vi "pruebaMaquinaEstados.vi"() -> ()   [LabVIEW 2016]
uses:
  Control 1.ctl
  <vilib>/userdefined/High Color/IMAQdx.ctl
  <vilib>/vision/driver/NI_Vision_Acquisition_Software.lvlib
panel:
  in  "Guardado":bool
  in  "D 4":i32
  in  "I 3":i32
  in  "I 2":i32
  in  "I 1":i32
  in  "D 3":i32
  in  "D 2":i32
  in  "D 1":i32
  in  "Movimiento de spot en x":ext(slide)=0.5255 scale=-10.0..10.0
  in  "Movimiento de spot en y":dbl(slide)=0.78 min=-10.0 max=10.0 scale=-10.0..10.0
  in  "Gráficas visibles":bool[](array[boolean])=[FALSE, FALSE, TRUE, FALSE, FALSE, FALSE]
  in  "Ver cámara":bool
  out "Image Pixels (U8)":u8[][](array[numeric])
  out "espectro aeereglo":dbl[][](array[numeric])
  in  "Cancel Button":bool
  in  "Guardar":bool=TRUE
  in  "valor delay":u32=300
  in  "tiempo de delay":u32=300
  out "Orden":T1(array[ring])=[enum."espejos", enum."voltaje", enum."polarizador", enum."potenciometro ", enum."CCD"]
  in  "Nombre  archivo":string="prueba0404"
  in  "stop medición":bool
  in  "stop":bool
  in  "Iniciar medición":bool
  out "Control de espejos":T2={"Movimiento de spot en y"=0.78, "Movimiento de spot en x"=0.5255, "tipo "=enum."barrido", "yFin"=0.82, "Paso"=0.01, "xFin"=0.5655} {"Movimiento de spot en x" scale=-10.0..10.0; "Movimiento de spot en y" min=-10.0 max=10.0 scale=-10.0..10.0}
  out "Config. voltaje y corriente":T3 {"Measurement Function (0:Voltage)" items=["Voltage", "Current", "Power"]; "Unit(V)" items=["V", "mV", "kV", "A", "mA"]; "Function(0:Voltage)" items=["Voltage", "Current"]}
  out "Laser":T4
  out "Config. fotodiodo y potenciometro":T5={"tiempo. lect."=300, "num. med"=20, "tiempo. lectura"=0, "average rate"=0, "Readout Config"="POW", "Tipo de Medición"=enum."Lockin", "usar multimetro"=FALSE}
  out "Control CCD":T6={"Numero de lecturas"=0, "tiempo de lectura (ms)"=100, "Exposure"=0.053229, "Valor Gamma"=1.0, "Ganancia"=33, "Opción"=enum."Espectro", "VISA resource name"="", "Enable Strobe (Disabled)"=FALSE} {"Ganancia" min=0 max=100; "Valor Gamma" min=1.0 max=2.2; "Exposure" min=5e-05 max=0.053229}
  out "config. Polarizador":T7={"pos inic"=0.0, "pos.final"=5.0, "incremento"=1.0, "velocidad"=0.0}
  in  "medir corriente":bool
  out "xsal":dbl=-0.20408163265306034
  out "ysal":dbl
  out "Ángulo del polarizador":dbl=5.000014648473263
  out "corriente":dbl
  out "voltaje":dbl
  out "temperatura":dbl
  out "corriente laser":dbl
  out "multimetro":dbl
  out "valor potenciometro":dbl=nan format="%^#_9e"
  out "LockIn":dbl=0.0003
  out "multímetro":T8
  out "Dr/r":T8
  out "espectro":T8={[0.0, 1.0, 2.0000073242366314, 3.0000073242366314, 4.000007324236631, 5.000014648473263], [0.0003, 0.0003, 0.0003, 0.0003, 0.0003, 0.0003]}
  out "I-V":cluster{dbl[], dbl[]}(graph)
  out "Gráfica general":T8={[0.0, 1.0, 2.0000073242366314, 3.0000073242366314, 4.000007324236631, 5.000014648473263], [0.0003, 0.0003, 0.0003, 0.0003, 0.0003, 0.0003]}
  out "Power meter":cluster{dbl[], dbl[]}(graph)
  out "Imágen":T9(plugin-control)
  in  "SerialNumber":string="55000538"
  # "Gráfica general"
  # "Gráfica potenciómetro"
  # "Gráfica I-V"
  # "Control espejos"
  # "Multímetro"
  # "División"
  # "Espectro"
  # "Amplificador Lock in"
  # "potenciometro"
  # "Espectro"
  # "Imágen"
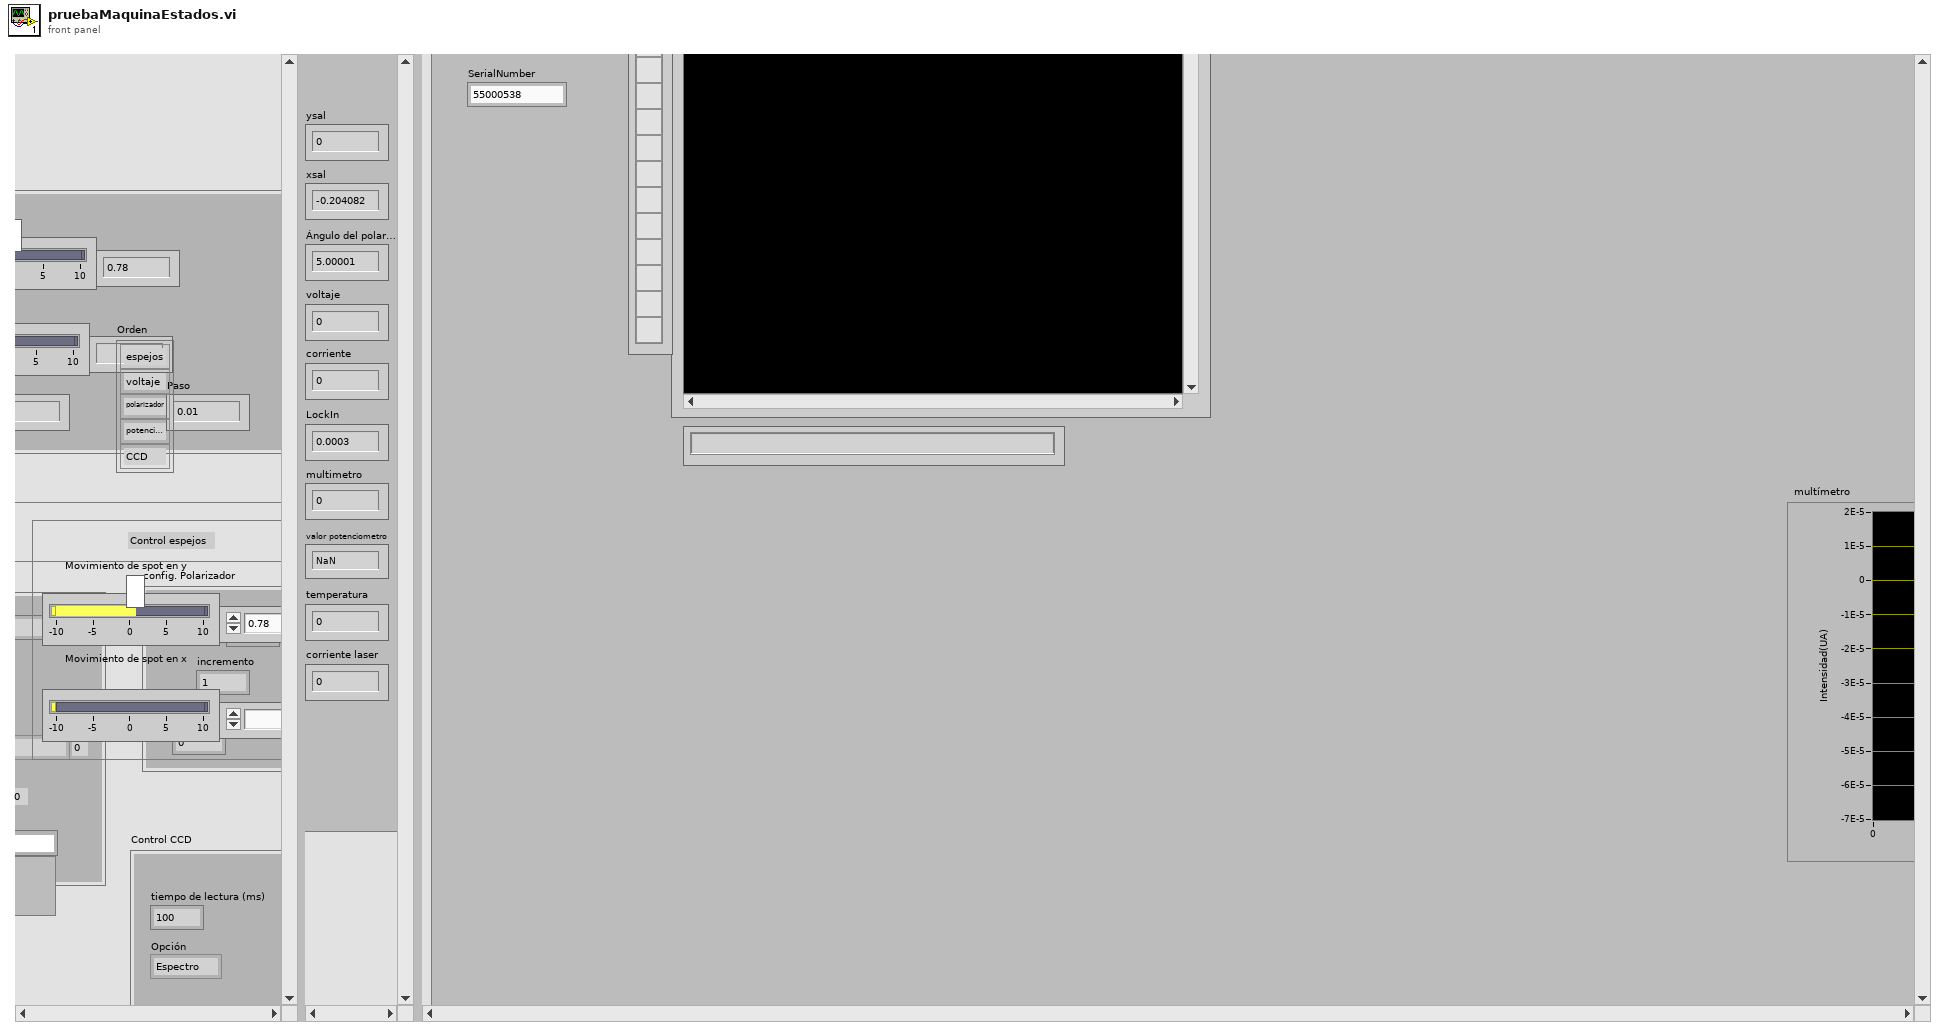
[diagram p1: front panel]
types:
  T1 = enum16{"espejos", "polarizador", "voltaje", "potenciometro ", "CCD", "lockin", "laser", "ninguno"}[]
  T2 = cluster{"Movimiento de spot en y":dbl, "Movimiento de spot en x":ext, "tipo ":enum16{"manual", "barrido"}, "yFin":dbl, "Paso":dbl, "xFin":dbl}
  T3 = cluster{"Voltaje inicial":dbl, "incremento":dbl, " voltaje final":dbl, "Function(0:Voltage)":u16, "Unit(V)":u16, "Measurement Function (0:Voltage)":u16, "VISA resource name":refnum<visa-resource-name>}
  T4 = cluster{"corriente inicial":dbl, "temperatura":dbl, "corriente final ":dbl, "incremento":dbl}
  T5 = cluster{"tiempo. lect.":i32, "num. med":i32, "tiempo. lectura":i32, "average rate":i32, "Readout Config":string, "Tipo de Medición":enum16{"Lockin", "Lockin-potenciometro", "Potenciometro"}, "usar multimetro":bool}
  T6 = cluster{"Numero de lecturas":i32, "tiempo de lectura (ms)":u32, "Exposure":dbl, "Valor Gamma":dbl, "Ganancia":i64, "Opción":enum16{"Espectro", "Imágen"}, "VISA resource name":refnum<visa-resource-name>, "Enable Strobe (Disabled)":bool}
  T7 = cluster{"pos inic":dbl, "pos.final":dbl, "incremento":dbl, "velocidad":dbl}
  T8 = typedef "Control 1.ctl" = cluster{dbl[], dbl[]}
  T9 = typedef "IMAQ Image.ctl" = refnum<image>
  T10 = typedef "IMAQdx.ctl" = refnum<k21>
  T11 = enum16{"Lockin", "Lockin-potenciometro", "Potenciometro"}
  T12 = enum16{"espejos", "polarizador", "voltaje", "potenciometro ", "CCD", "lockin", "laser", "ninguno"}
  T13 = cluster{"Global Rectangle":i32[], "Contours":cluster{"Contour Type":u32, "ROI Type":u32, "Points":i32[]}[]}
  T14 = cluster{"a0":dbl[][], "a1":dbl[][][], "a2":dbl[][][][], "a3":dbl[][][][][]}
  T15 = cluster{"Wavelength (nm)":dbl[], "arreglo promedio":dbl[]}
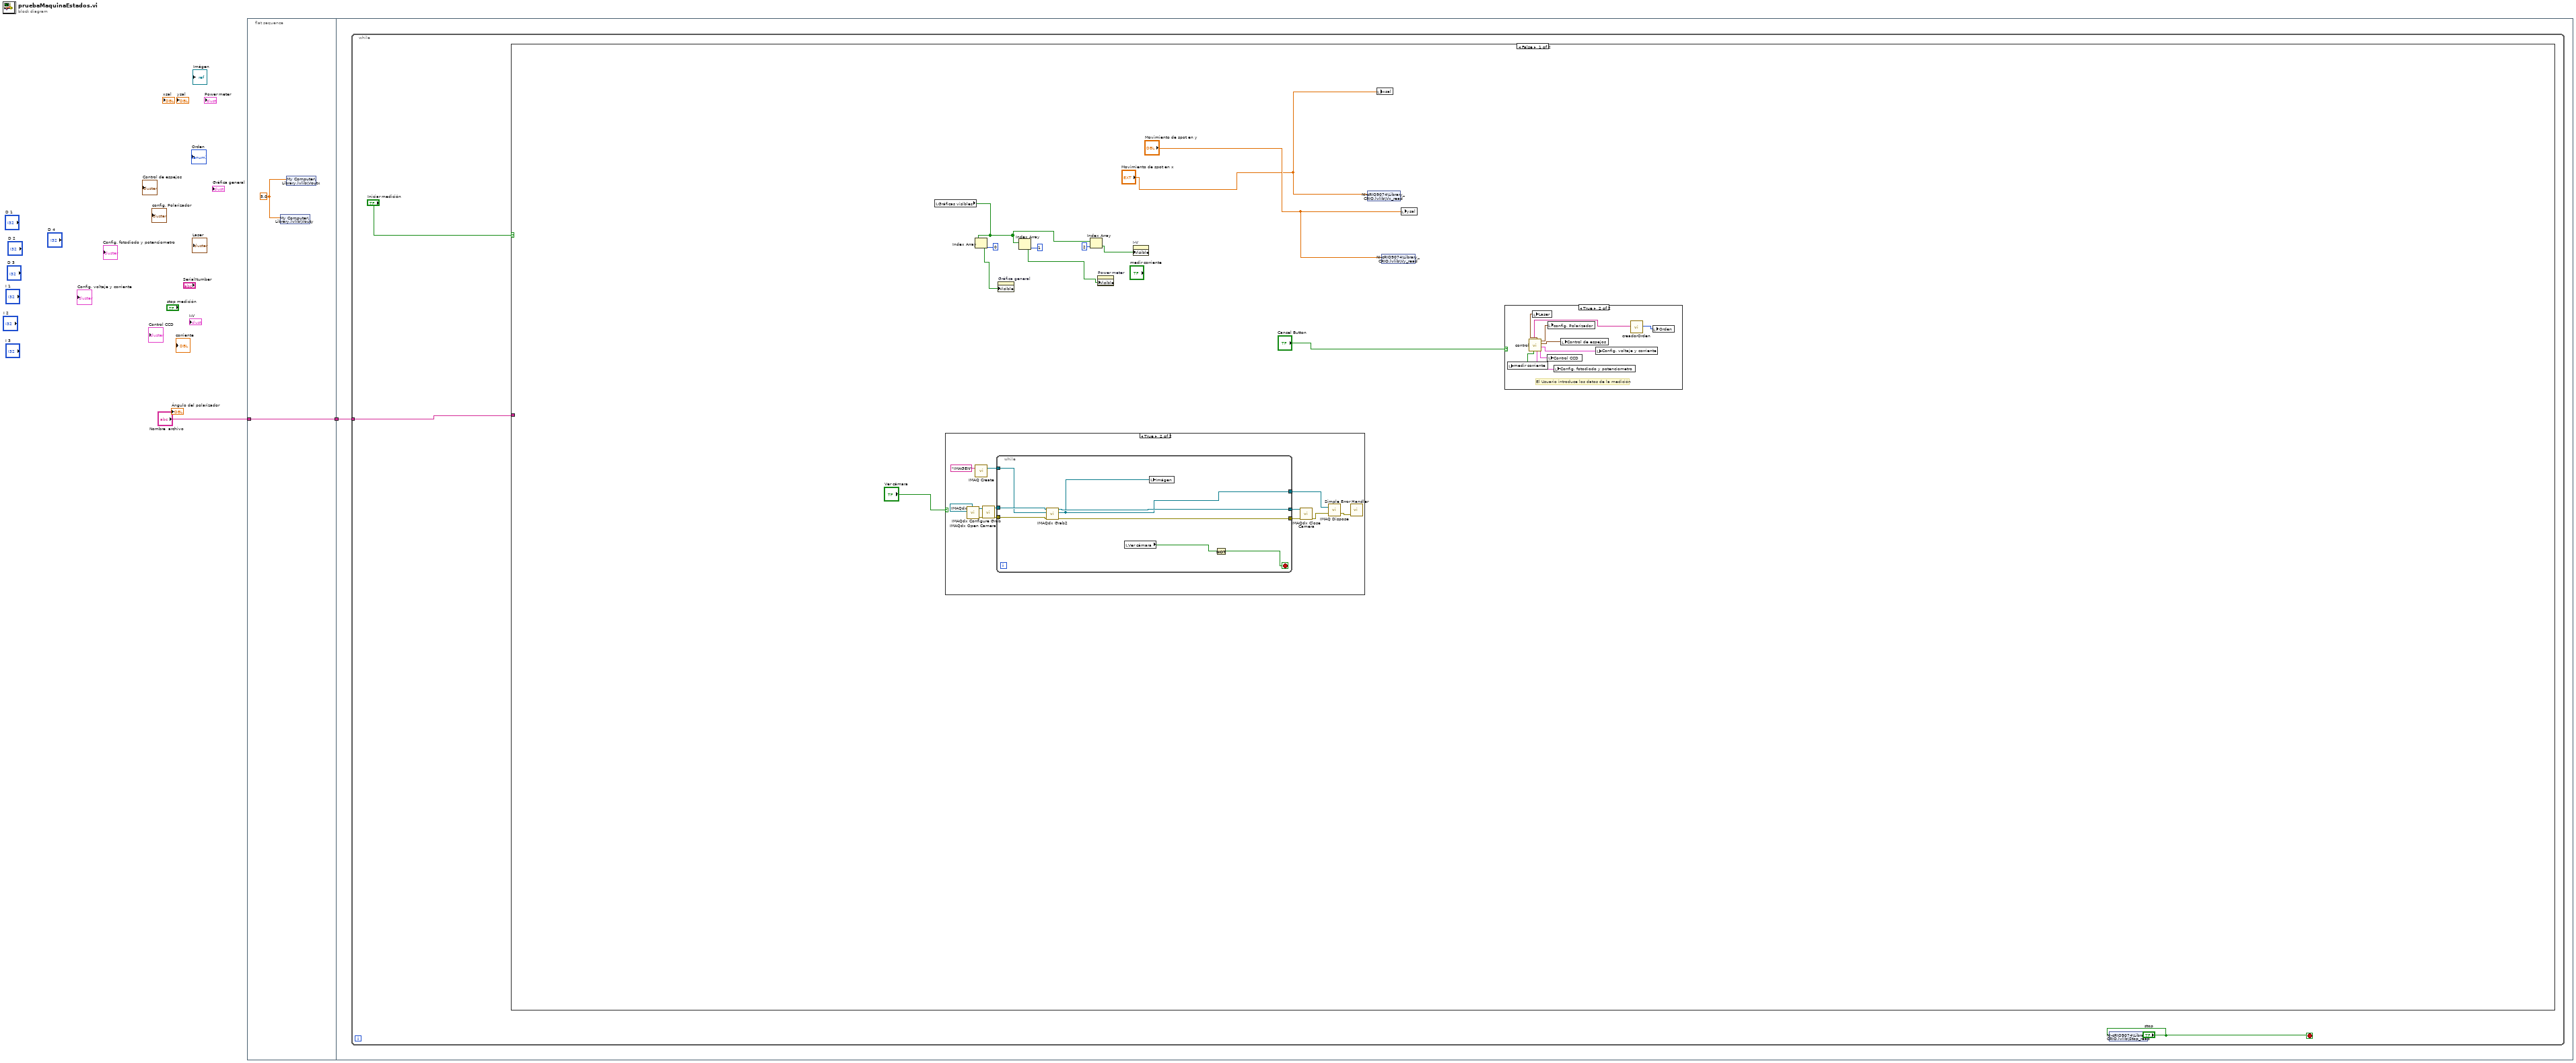
[diagram p0: block diagram]
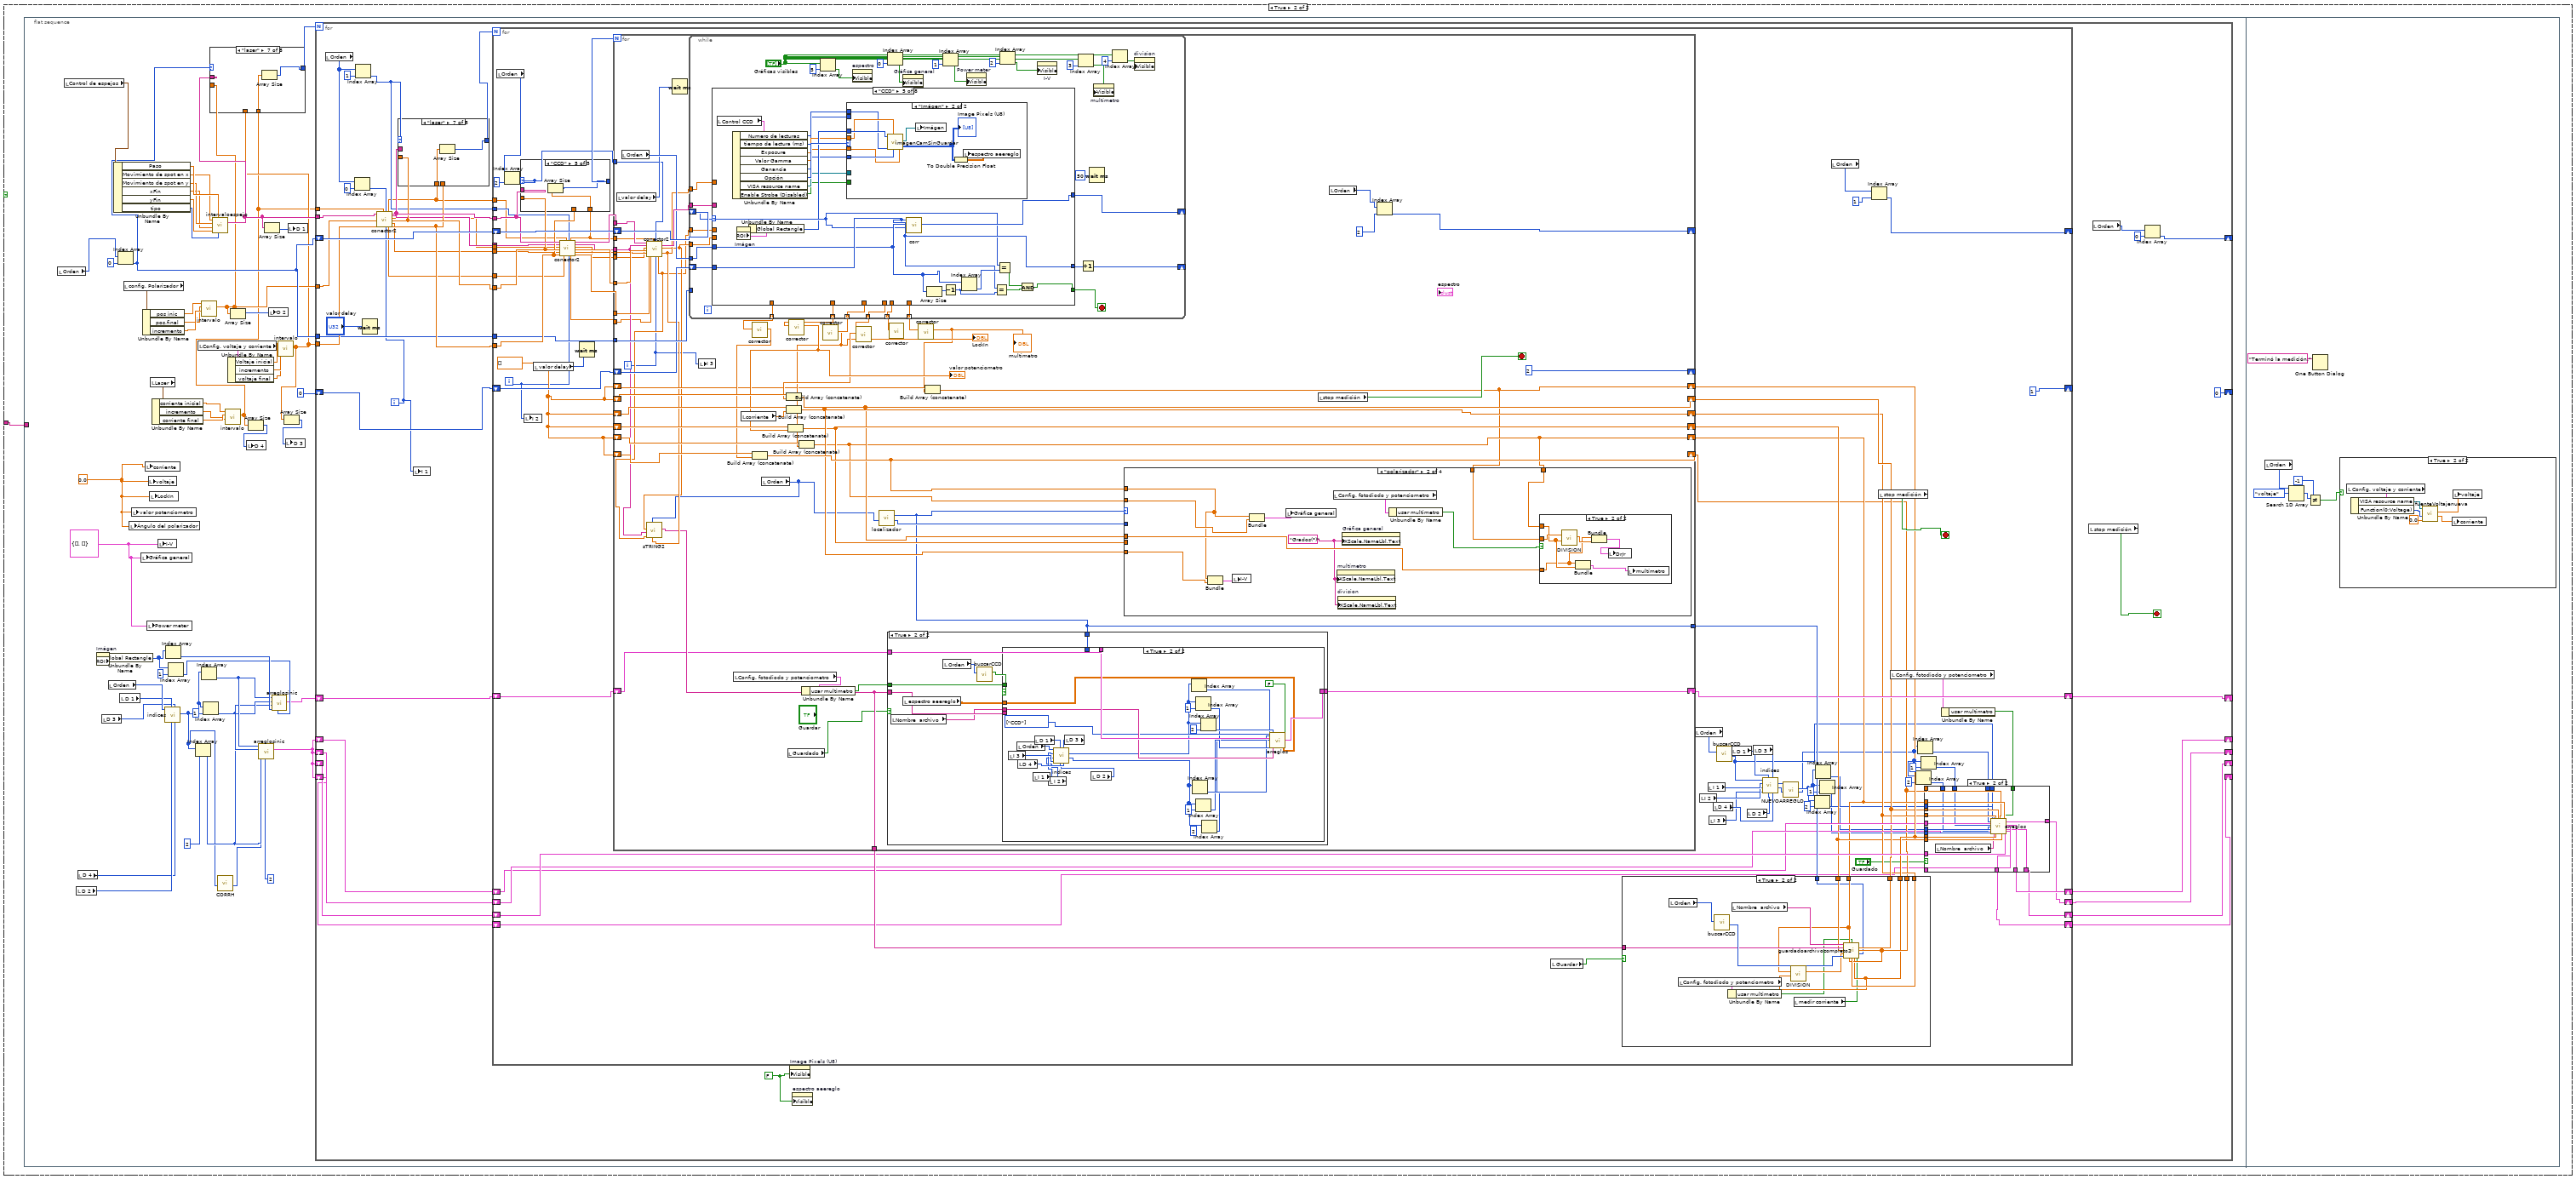
[diagram p4: hidden frame]
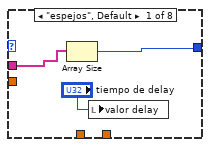
[diagram p5: hidden frame]
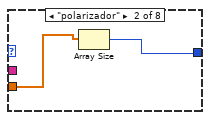
[diagram p6: hidden frame]
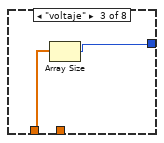
[diagram p7: hidden frame]
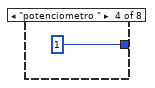
[diagram p8: hidden frame]
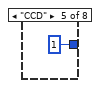
[diagram p9: hidden frame]
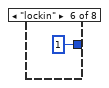
[diagram p10: hidden frame]
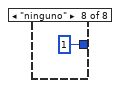
[diagram p11: hidden frame]
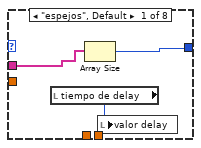
[diagram p12: hidden frame]
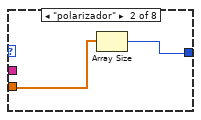
[diagram p13: hidden frame]
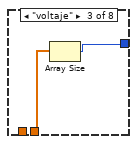
[diagram p14: hidden frame]
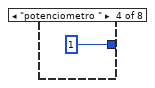
[diagram p15: hidden frame]
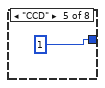
[diagram p16: hidden frame]
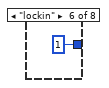
[diagram p17: hidden frame]
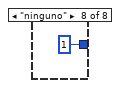
[diagram p18: hidden frame]
diagram:
  n1 = flat-sequence {
    tunnel: "Nombre  archivo" -> [w3]
    tunnel: [w3] -> w1
    tunnel: w1 -> [w5]
    frame #0 {
      w4 = 5.0
      n2 = shared-variable "My Computer\\Library.lvlib\\Vouty"(w4) -> ()  [unwired: 1 in, 1 out]
      n3 = shared-variable "My Computer\\Library.lvlib\\Voutx"(w4) -> ()  [unwired: 1 in, 1 out]
    }
    frame #1 {
      n4 = while {
        tunnel: w5 -> [w6]
        stop <- "stop" stop-if-true
        n5 = case shown="False" "Iniciar medición" {
          tunnel: w6 -> [_ w49]
          frame False {
            n6 = local read "Gráficas visibles"() -> (w16:bool[])
            n7 = case shown="True" "Ver cámara" {
              frame False {
              }
              frame True {
                n8 = call <vilib>:"IMAQdx Open Camera.vi"("Session In"=T10 "cam4") -> ("error out"=w31:errorcluster, "Session Out"=w30:T10)  [unwired: 9 in]
                n9 = call "IMAQ Create"("Image Name"="IMAGEN") -> ("New Image"=w27:T9)  [unwired: 4 in, 1 out]
                n10 = call <vilib>:"IMAQdx Configure Grab.vi"("error in"=w31, "Session In"=w30) -> ("error out"=w28:errorcluster, "Session Out"=w29:T10)  [unwired: 8 in]
                n11 = while {
                  tunnel: w29 -> [w39]
                  tunnel: w28 -> [w38]
                  tunnel: w27 -> [w37]
                  tunnel: [w36] -> w25
                  tunnel: [w35] -> w24
                  tunnel: [w32] -> w22
                  stop <- w33 stop-if-true
                  n12 = call <vilib>:"IMAQdx Grab2.vi"("error in"=w38, "Image In"=w37, "Session In"=w39) -> ("error out"=w35:errorcluster, "Image Out"=w32:T9, "Session Out"=w36:T10)  [unwired: 5 in, 1 out]
                  n13 = local read "Ver cámara"() -> (w34:bool)
                  n14 = local write "Imágen"(w32) -> ()
                  n15 = Not(x=w34) -> (.not. x?=w33:bool)
                }
                n16 = call <vilib>:"IMAQdx Close Camera.vi"("error in"=w24, "Session In"=w25) -> ("error out"=w23:errorcluster)  [unwired: 9 in]
                n17 = call "IMAQ Dispose"("Image"=w22, "error in (no error)"=w23) -> ("error out"=w21:errorcluster)  [unwired: 4 in]
                n18 = call <vilib>:"Simple Error Handler.vi"("error in (no error)"=w21) -> ()  [unwired: 4 in, 5 out]
              }
            }
            n19 = Index Array(array=w16, index=0) -> (element=w15:bool)
            n20 = property on="Gráfica general" class="XYGraph (strict)"("Visible"=w15) -> ()  [unwired: 2 in, 2 out]
            n21 = Index Array(array=w16, index=1) -> (element=w14:bool)
            n22 = Index Array(array=w16, index=2) -> (element=w13:bool)
            n23 = property on="Power meter" class="XYGraph (strict)"("Visible"=w14) -> ()  [unwired: 2 in, 2 out]
            n24 = property on="I-V" class="XYGraph (strict)"("Visible"=w13) -> ()  [unwired: 2 in, 2 out]
            n25 = shared-variable "NI-cRIO9074\\Library_CRIO.lvlib\\Vx_read"("Movimiento de spot en x") -> ()  [unwired: 1 in, 1 out]
            n26 = local write "xsal"("Movimiento de spot en x") -> ()
            n27 = shared-variable "NI-cRIO9074\\Library_CRIO.lvlib\\Vy_read"("Movimiento de spot en y") -> ()  [unwired: 1 in, 1 out]
            n28 = local write "ysal"("Movimiento de spot en y") -> ()
            n29 = case shown="True" "Cancel Button" {
              frame False {
              }
              frame True {
                # "El Usuario introduce los datos de la medición"
                n30 = call "control.vi"() -> ("Control CCD"=w45:T6, "Config. voltaje y corriente"=w46:T3, "Control de espejos"=w47:T2, "config. Polarizador"=w48:T7, "Config. fotodiodo y potenciometro"=w44:T5, "Laser"=w43:T4, "corriente"=w40:bool, "dispositivos"=w42:string[])  [unwired: 4 in]
                n31 = local write "medir corriente"(w40) -> ()
                n32 = local write "Laser"(w43) -> ()
                n33 = local write "Control CCD"(w45) -> ()
                n34 = local write "config. Polarizador"(w48) -> ()
                n35 = local write "Config. fotodiodo y potenciometro"(w44) -> ()
                n36 = local write "Control de espejos"(w47) -> ()
                n37 = local write "Config. voltaje y corriente"(w46) -> ()
                n38 = call "creadorOrden.vi"("Array"=w42) -> ("Array 2"=w41:T1)  [unwired: 10 in]
                n39 = local write "Orden"(w41) -> ()
              }
            }
          }
          frame True {
            n40 = flat-sequence {
              tunnel: w49 -> [_]
              frame #0 {
                w92 = cluster{dbl[], dbl[]} {[], []} ("I-V")
                w93 = 0.0
                n41 = local read "Orden"() -> (w78:T1)
                n42 = local read "Control de espejos"() -> (w91:T2)
                n43 = local read "D 2"() -> (w71:i32)
                n44 = local read "D 4"() -> (w65:i32)
                n45 = property on="Imágen" class="ImageControl"() -> ("ROI"=w62:T13)  [unwired: 2 in, 2 out]
                n46 = Unbundle By Name(w62) -> ("Global Rectangle"=w60:i32[])
                n47 = local read "D 3"() -> (w67:i32)
                n48 = local read "Orden"() -> (w75:T1)
                n49 = Unbundle By Name(w91) -> ("Paso"=w90:dbl, "Movimiento de spot en x"=w89:ext, "Movimiento de spot en y"=w88:dbl, "xFin"=w87:dbl, "yFin"=w86:dbl, "tipo"=w85:enum16{"manual", "barrido"})
                n50 = Index Array(array=w78, index=0) -> (element=w84:T12)
                n51 = local read "D 1"() -> (w74:i32)
                n52 = local read "config. Polarizador"() -> (w103:T7)
                n53 = local write "Ángulo del polarizador"(w93) -> ()
                n54 = local write "valor potenciometro"(w93) -> ()
                n55 = local write "Gráfica general"(w92) -> ()
                n56 = Unbundle By Name(w103) -> ("pos inic"=w102:dbl, "pos.final"=w100:dbl, "incremento"=w101:dbl)
                n57 = local write "corriente"(w93) -> ()
                n58 = local write "Power meter"(w92) -> ()
                n59 = local write "voltaje"(w93) -> ()
                n60 = local write "LockIn"(w93) -> ()
                n61 = local read "Laser"() -> (w82:T4)
                n62 = Unbundle By Name(w82) -> ("corriente inicial"=w81:dbl, "incremento"=w79:dbl, "corriente final"=w80:dbl)
                n63 = local write "I-V"(w92) -> ()
                n64 = call "indices.vi"("corriente laser"=w65, "voltaje"=w67, "polarizador"=w71, "espejo"=w74, "Orden"=w75) -> ("dimensiones"=w53:i32[])  [unwired: 5 in, 1 out]
                n65 = Index Array(array=w60) -> (element=w61:i32)  [unwired: 1 in]
                n66 = Index Array(array=w60, index=1) -> (element=w58:i32)
                n67 = Index Array(array=w53, index=2) -> (element=w55:i32)
                n68 = local read "Config. voltaje y corriente"() -> (w99:T3)
                n69 = call "intervalo.vi"("incremento"=w101, "fin"=w100, "inicio"=w102) -> ("Array"=w73:dbl[])  [unwired: 8 in]
                n70 = Index Array(array=w53) -> (element=w57:i32)  [unwired: 1 in]
                n71 = Index Array(array=w53, index=1) -> (element=w56:i32)
                n72 = call "intervaloespejo.vi"("tipo"=w85, "intervalo"=w90, "fin y"=w86, "fin x"=w87, "inicio y"=w88, "inicio x"=w89) -> ("salida"=w77:string[])  [unwired: 5 in]
                n73 = call "CORRH.vi"("Array"=w53) -> ("element"=w52:i32)  [unwired: 10 in]
                n74 = call "intervalo.vi"("incremento"=w79, "fin"=w80, "inicio"=w81) -> ("Array"=w68:dbl[])  [unwired: 8 in]
                n75 = Unbundle By Name(w99) -> ("Voltaje inicial"=w98:dbl, "incremento"=w97:dbl, "voltaje final"=w96:dbl)
                n76 = Array Size(array=w73) -> (size(s)=w72:i32)
                n77 = Array Size(array=w68) -> (size(s)=w66:i32)
                n78 = local write "D 4"(w66) -> ()
                n79 = call "arreglosinic.vi"("dimension adqy"=2, "dimension adqx"=w52, "DISPLONG 3"=w55, "DISPLONG 2"=w56, "DISPLONG 1"=w57) -> ("output cluster"=w50:T14)  [unwired: 5 in]
                n80 = Array Size(array=w77) -> (size(s)=w76:i32)
                n81 = local write "D 2"(w72) -> ()
                n82 = call "arreglosinic.vi"("dimension adqy"=w58, "dimension adqx"=w61, "DISPLONG 3"=w55, "DISPLONG 2"=w56, "DISPLONG 1"=w57) -> ("output cluster"=w51:T14)  [unwired: 5 in]
                n83 = call "intervalo.vi"("incremento"=w97, "fin"=w96, "inicio"=w98) -> ("Array"=w70:dbl[])  [unwired: 8 in]
                n84 = case shown="\"laser\"" w84 {
                  tunnel: [w105 w107 w109 1 1 1 w115 1] -> w94
                  tunnel: w77 -> [w106 _ _ _ _ _ _ _]
                  tunnel: w73 -> [_ w108 _ _ _ _ _ _]
                  tunnel: w70 -> [_ _ w110 _ _ _ _ _]
                  tunnel: w68 -> [_ _ _ _ _ _ w114 _]
                  frame "espejos", Default {
                    n85 = Array Size(array=w106) -> (size(s)=w105:i32)
                    n86 = local write "valor delay"("tiempo de delay") -> ()
                  }
                  frame "polarizador" {
                    n87 = Array Size(array=w108) -> (size(s)=w107:i32)
                  }
                  frame "voltaje" {
                    n88 = Array Size(array=w110) -> (size(s)=w109:i32)
                  }
                  frame "potenciometro " {
                  }
                  frame "CCD" {
                  }
                  frame "lockin" {
                  }
                  frame "laser" {
                    n89 = Array Size(array=w114) -> (size(s)=w115:i32)
                  }
                  frame "ninguno" {
                  }
                }
                n90 = Array Size(array=w70) -> (size(s)=w69:i32)
                n91 = local write "D 3"(w69) -> ()
                n92 = local write "D 1"(w76) -> ()
                n93 = for {
                  N: w94 -> [_]
                  tunnel: w77 -> [w132]
                  shift-right: [w135] -> _
                  shift-left: w84 -> [w155]
                  tunnel: w73 -> [w152]
                  tunnel: w70 -> [w151]
                  tunnel: w84 -> [w144]
                  shift-right: [0] -> _
                  shift-left: 0 -> [w133]
                  tunnel: w68 -> [w131]
                  shift-right: [w125] -> _
                  shift-left: w51 -> [w126]
                  shift-right: [w121] -> _
                  shift-left: w50 -> [w124]
                  shift-right: [w120] -> _
                  shift-left: w50 -> [w123]
                  shift-right: [w119] -> _
                  shift-left: w50 -> [w122]
                  shift-right: [w117] -> _
                  shift-left: w50 -> [w118]
                  i -> [w127]
                  stop <- w137 stop-if-true
                  w128 = FALSE ("Visible")
                  n94 = local read "Orden"() -> (w143:T1)
                  n95 = Index Array(array=w143, index=0) -> (element=w138:T12)
                  n96 = Index Array(array=w143, index=1) -> (element=w141:T12)
                  n97 = Wait (ms)(milliseconds to wait="valor delay") -> ()  [unwired: 1 out]
                  n98 = call "conector2.vi"("salida"=w132, "polarizador"=w152, "voltaje"=w151, "corrientes"=w131, "Enum"=w138, "Indice"=w127) -> ("corrientes salida"=w129:dbl[], "VoltajeEnt 2"=w145:dbl, "salida 2"=w150:string[], "Salida ent 2"=w147:string, "corriente salida"=w130:dbl, "polarizador 2"=w149:dbl[], "Polarizador"=w146:dbl, "voltaje 2"=w148:dbl[])  [unwired: 6 in]
                  n99 = case shown="\"laser\"" w141 {
                    tunnel: [w157 w159 w161 1 1 1 w166 1] -> w154
                    tunnel: w150 -> [w158 _ _ _ _ _ _ _]
                    tunnel: w149 -> [_ w160 _ _ _ _ _ _]
                    tunnel: w148 -> [_ _ w162 _ _ _ _ _]
                    tunnel: w129 -> [_ _ _ _ _ _ w167 _]
                    frame "espejos", Default {
                      n100 = local read "tiempo de delay"() -> (w156:u32)
                      n101 = Array Size(array=w158) -> (size(s)=w157:i32)
                      n102 = local write "valor delay"(w156) -> ()
                    }
                    frame "polarizador" {
                      n103 = Array Size(array=w160) -> (size(s)=w159:i32)
                    }
                    frame "voltaje" {
                      n104 = Array Size(array=w162) -> (size(s)=w161:i32)
                    }
                    frame "potenciometro " {
                    }
                    frame "CCD" {
                    }
                    frame "lockin" {
                    }
                    frame "laser" {
                      n105 = Array Size(array=w167) -> (size(s)=w166:i32)
                    }
                    frame "ninguno" {
                    }
                  }
                  n106 = local write "I 1"(w127) -> ()
                  n107 = for {
                    N: w154 -> [_]
                    tunnel: w150 -> [w238]
                    shift-right: [w223] -> _
                    shift-left: w155 -> [w245]
                    tunnel: w149 -> [w237]
                    tunnel: w148 -> [w236]
                    tunnel: w147 -> [w235]
                    tunnel: w146 -> [w234]
                    tunnel: w145 -> [w233]
                    tunnel: w144 -> [w232]
                    tunnel: w141 -> [w225]
                    shift-right: [1] -> _
                    shift-left: w133 -> [w220]
                    tunnel: w130 -> [w218]
                    tunnel: w129 -> [w217]
                    shift-right: [w209] -> w125
                    shift-left: w126 -> [w210]
                    shift-right: [w208] -> w121
                    shift-left: w124 -> [w202]
                    shift-right: [w207] -> w120
                    shift-left: w123 -> [w203]
                    shift-right: [w206] -> w119
                    shift-left: w122 -> [w205]
                    shift-right: [w172] -> w117
                    shift-left: w118 -> [w173]
                    i -> [w211]
                    stop <- w224 stop-if-true
                    w219 = dbl[] []
                    n108 = local read "Orden"() -> (w243:T1)
                    n109 = Index Array(array=w243, index=2) -> (element=w231:T12)
                    n110 = local write "I 2"(w211) -> ()
                    n111 = local read "valor delay"() -> (w230:u32)
                    n112 = call "conector2.vi"("salida"=w238, "Salida ent"=w235, "corriente entrada"=w218, "polarizador"=w237, "Polarizadorent"=w234, "voltaje"=w236, "VoltajeEnt"=w233, "corrientes"=w217, "Enum"=w225, "Indice"=w211) -> ("corrientes salida"=w216:dbl[], "VoltajeEnt 2"=w228:dbl, "salida 2"=w241:string[], "Salida ent 2"=w227:string, "corriente salida"=w215:dbl, "polarizador 2"=w240:dbl[], "Polarizador"=w226:dbl, "voltaje 2"=w239:dbl[])  [unwired: 2 in]
                    n113 = case shown="\"CCD\"" w231 {
                      tunnel: [w289 w291 w293 1 w297] -> w244
                      tunnel: w238 -> [w290 _ _ _ _]
                      tunnel: w237 -> [_ w292 _ _ _]
                      tunnel: w236 -> [_ _ w294 _ _]
                      tunnel: w216 -> [_ _ _ _ w296]
                      frame "espejos", Default {
                        n114 = local read "tiempo de delay"() -> (w288:u32)
                        n115 = local write "valor delay"(w288) -> ()
                        n116 = Array Size(array=w290) -> (size(s)=w289:i32)
                      }
                      frame "polarizador" {
                        n117 = Array Size(array=w292) -> (size(s)=w291:i32)
                      }
                      frame "voltaje" {
                        n118 = Array Size(array=w294) -> (size(s)=w293:i32)
                      }
                      frame "potenciometro " {
                      }
                      frame "CCD" {
                        n119 = Array Size(array=w296) -> (size(s)=w297:i32)
                      }
                    }
                    n120 = Wait (ms)(milliseconds to wait=w230) -> ()  [unwired: 1 out]
                    n121 = for {
                      N: w244 -> [_]
                      shift-right: [w324] -> _
                      shift-left: w245 -> [w354]
                      tunnel: w241 -> [w342]
                      tunnel: w240 -> [w341]
                      tunnel: w239 -> [w340]
                      shift-right: [w313] -> w201
                      shift-left: w219 -> [w353]
                      shift-right: [w331] -> w200
                      shift-left: w219 -> [w352]
                      shift-right: [w330] -> w199
                      shift-left: w219 -> [w351]
                      shift-right: [w312] -> w198
                      shift-left: w219 -> [w350]
                      tunnel: w228 -> [w307]
                      tunnel: w226 -> [w338]
                      tunnel: w227 -> [w315]
                      tunnel: w232 -> [w336]
                      tunnel: w231 -> [w327]
                      shift-right: [w332] -> w197
                      shift-left: w219 -> [w334]
                      shift-right: [2] -> _
                      shift-left: w220 -> [w322]
                      shift-right: [w311] -> w204
                      shift-left: w219 -> [w320]
                      tunnel: w216 -> [w318]
                      tunnel: w215 -> [w317]
                      tunnel: [w304] -> w213
                      tunnel: [w303] -> w212
                      shift-right: [w299] -> w209
                      shift-left: w210 -> [w300]
                      i -> [w301]
                      stop <- w326 stop-if-true
                      n122 = local read "valor delay"() -> (w329:u32)
                      n123 = local read "Orden"() -> (w337:T1)
                      n124 = call "conector2.vi"("salida"=w342, "Salida ent"=w315, "corriente entrada"=w317, "polarizador"=w341, "Polarizadorent"=w338, "voltaje"=w340, "VoltajeEnt"=w307, "corrientes"=w318, "Enum"=w327, "Indice"=w301) -> ("VoltajeEnt 2"=w308:dbl, "Salida ent 2"=w339:string, "corriente salida"=w314:dbl, "Polarizador"=w316:dbl)  [unwired: 2 in, 4 out]
                      n125 = Wait (ms)(milliseconds to wait=w329) -> ()  [unwired: 1 out]
                      n126 = while {
                        shift-right: [w453] -> _
                        shift-left: w354 -> [w459]
                        tunnel: w339 -> [w458]
                        tunnel: w316 -> [w451]
                        tunnel: w308 -> [w449]
                        tunnel: [w448] -> w346 mode=indexing
                        tunnel: [w447] -> w344 mode=indexing
                        tunnel: [w445] -> w347 mode=indexing
                        tunnel: [w444] -> w348 mode=indexing
                        tunnel: w337 -> [w456]
                        tunnel: w336 -> [_]
                        tunnel: [w450] -> w335 mode=indexing
                        shift-right: [w455] -> _
                        shift-left: w322 -> [w457]
                        tunnel: [w446] -> w321 mode=indexing
                        tunnel: w314 -> [w443]
                        stop <- w452 stop-if-true
                        n127 = case shown="\"CCD\"" w459 {
                          selector: w459 -> [w470 w485 w502 w518 w538 w573 w587 w598]
                          tunnel: w458 -> [w479 _ _ _ _ _ _ _]
                          tunnel: w457 -> [w469 w484 w500 w519 w540 w574 w589 w599]
                          tunnel: w456 -> [w471 w483 w503 w517 w539 w572 w588 w597]
                          tunnel: [w469 w484 w500 w519 w540 w574 w589 w599] -> w454
                          tunnel: [w468 w486 w499 w521 w542 w576 w591 w601] -> w453
                          tunnel: [w467 w487 w501 w520 w541 w575 w590 w600] -> w452
                          tunnel: w451 -> [_ w481 _ _ _ _ _ _]
                          tunnel: [_ w480 _ _ _ _ _ _] -> w450
                          tunnel: w449 -> [_ _ w496 _ _ _ _ _]
                          tunnel: [_ _ w495 _ _ _ _ _] -> w448
                          tunnel: [_ _ w494 _ _ _ _ _] -> w447
                          tunnel: [_ _ _ w510 _ w566 _ _] -> w446
                          tunnel: [_ _ _ _ _ w565 _ _] -> w445
                          tunnel: [_ _ _ w509 _ _ _ _] -> w444
                          tunnel: w443 -> [_ _ _ _ _ _ w584 _]
                          frame "espejos", Default {
                            n128 = call "controlespejo.vi"("cadena entrada"=w479) -> ("x"=w478:dbl, "y"=w477:dbl)  [unwired: 9 in]
                            n129 = local write "ysal"(w477) -> ()
                            n130 = local write "xsal"(w478) -> ()
                            n131 = call "corr.vi"("Enum"=w470, "Orden"=w471, "Numeric"=w469) -> ("Enum 2"=w468:T12)  [unwired: 8 in]
                            n132 = Array Size(array=w471) -> (size(s)=w476:i32)
                            n133 = Decrement(x=w476) -> (x-1=w472:i32)
                            n134 = Index Array(array=w471, index=w472) -> (element=w475:T12)
                            n135 = Equal?(x=w469, y=w472) -> (x = y?=w474:bool)
                            n136 = Equal?(x=w470, y=w475) -> (x = y?=w473:bool)
                            n137 = And(x=w473, y=w474) -> (x .and. y?=w467:bool)
                          }
                          frame "polarizador" {
                            n138 = local read "SerialNumber"() -> (w482:string)
                            n139 = call "pol2.vi"("SerialNumber"=w482, "position"=w481) -> ("GetPositionCounter"=w480:dbl)  [unwired: 9 in]
                            n140 = local write "Ángulo del polarizador"(w480) -> ()
                            n141 = call "corr.vi"("Enum"=w485, "Orden"=w483, "Numeric"=w484) -> ("Enum 2"=w486:T12)  [unwired: 8 in]
                            n142 = Array Size(array=w483) -> (size(s)=w492:i32)
                            n143 = Decrement(x=w492) -> (x-1=w488:i32)
                            n144 = Index Array(array=w483, index=w488) -> (element=w491:T12)
                            n145 = Equal?(x=w484, y=w488) -> (x = y?=w490:bool)
                            n146 = Equal?(x=w485, y=w491) -> (x = y?=w489:bool)
                            n147 = And(x=w489, y=w490) -> (x .and. y?=w487:bool)
                          }
                          frame "voltaje" {
                            n148 = local read "Config. voltaje y corriente"() -> (w498:T3)
                            n149 = Unbundle By Name(w498) -> ("Function(0:Voltage)"=w497:u16)  [unwired: 1 out]
                            n150 = call "fuenteVoltajenueva.vi"("entrada"=w496, "Source Mode  (0: Voltage)"=w497, "VISA resource name"=refnum<visa-resource-name> "USB0::0x05E6::0x2450::04435662::INSTR") -> ("CORRIENTE"=w494:dbl, "VOLTAJE"=w495:dbl)  [unwired: 7 in]
                            "voltaje" <- w495
                            n151 = local write "corriente"(w494) -> ()
                            n152 = call "corr.vi"("Enum"=w502, "Orden"=w503, "Numeric"=w500) -> ("Enum 2"=w499:T12)  [unwired: 8 in]
                            n153 = Array Size(array=w503) -> (size(s)=w508:i32)
                            n154 = Decrement(x=w508) -> (x-1=w504:i32)
                            n155 = Index Array(array=w503, index=w504) -> (element=w507:T12)
                            n156 = Equal?(x=w500, y=w504) -> (x = y?=w506:bool)
                            n157 = Equal?(x=w502, y=w507) -> (x = y?=w505:bool)
                            n158 = And(x=w505, y=w506) -> (x .and. y?=w501:bool)
                          }
                          frame "potenciometro " {
                            n159 = local read "Config. fotodiodo y potenciometro"() -> (w516:T5)
                            n160 = Unbundle By Name(w516) -> ("tiempo. lectura"=w512:i32, "average rate"=w513:i32, "Readout Config"=w514:string, "usar multimetro"=w515:bool)
                            n161 = call "controllockin.vi"("usar multimetro"=w515, "Enum"=T11."Potenciometro", "Readout Config"=w514, "average rate"=w513, "tiempo lecturas potenciomtro"=w512) -> ("multimetro"=w510:dbl, "valor potenciometro"=w509:dbl)  [unwired: 4 in, 1 out]
                            n162 = call "corr.vi"("Enum"=w518, "Orden"=w517, "Numeric"=w519) -> ("Enum 2"=w521:T12)  [unwired: 8 in]
                            n163 = Array Size(array=w517) -> (size(s)=w522:i32)
                            n164 = Decrement(x=w522) -> (x-1=w526:i32)
                            n165 = Index Array(array=w517, index=w526) -> (element=w523:T12)
                            n166 = Equal?(x=w519, y=w526) -> (x = y?=w524:bool)
                            n167 = Equal?(x=w518, y=w523) -> (x = y?=w525:bool)
                            n168 = And(x=w525, y=w524) -> (x .and. y?=w520:bool)
                          }
                          frame "CCD" {
                            n169 = local read "Control CCD"() -> (w537:T6)
                            n170 = Unbundle By Name(w537) -> ("Numero de lecturas"=w528:i32, "tiempo de lectura (ms)"=w530:u32, "Exposure"=w533:dbl, "Valor Gamma"=w531:dbl, "Ganancia"=w532:i64, "Opción"=w536:enum16{"Espectro", "Imágen"}, "VISA resource name"=w529:refnum<visa-resource-name>, "Enable Strobe (Disabled)"=w527:bool)
                            n171 = property on="Imágen" class="ImageControl"() -> ("ROI"=w535:T13)  [unwired: 2 in, 2 out]
                            n172 = Unbundle By Name(w535) -> ("Global Rectangle"=w534:i32[])
                            n173 = case shown="\"Imágen\"" w536 {
                              tunnel: w534 -> [_ w564]
                              tunnel: w533 -> [_ w563]
                              tunnel: w532 -> [_ w562]
                              tunnel: w531 -> [_ w561]
                              tunnel: w530 -> [w554 w560]
                              tunnel: w529 -> [w556 _]
                              tunnel: w528 -> [w555 _]
                              tunnel: w527 -> [w553 _]
                              frame "Espectro", Default {
                                n174 = call "espectroCCD.vi"("Enable Strobe (Disabled)"=w553, "tiempo de lectura (ms)"=w554, "Numero de lecturas"=w555, "VISA resource name"=w556) -> ("arreglo promedio"=w550:dbl[], "Wavelength (nm)"=w551:dbl[])  [unwired: 6 in]
                                n175 = Build Array(w551, w550) -> (w552:dbl[][])
                                n176 = Bundle("Wavelength (nm)"=w551, "arreglo promedio"=w550) -> (w549:T15)  [unwired: 1 in]
                                n177 = Transpose 2D Array(2D array=w552) -> (transposed array=→"espectro aeereglo":dbl[][])
                                n178 = local write "espectro"(w549) -> ()
                              }
                              frame "Imágen" {
                                n179 = call "imagenCamSinGuardar.vi"("Valor Gamma"=w561, "Ganancia"=w562, "Exposure"=w563, "tiempo de exposición (ms)"=w560, "Optional Rectangle"=w564) -> ("Image Pixels (U8)"=w559:u8[][], "Image"=w557:T9)  [unwired: 5 in]
                                "Image Pixels (U8)" <- w559
                                n180 = local write "Imágen"(w557) -> ()
                                n181 = To Double Precision Float(number=w559) -> (double precision float=w558:dbl[][])
                                n182 = local write "espectro aeereglo"(w558) -> ()
                              }
                            }
                            n183 = call "corr.vi"("Enum"=w538, "Orden"=w539, "Numeric"=w540) -> ("Enum 2"=w542:T12)  [unwired: 8 in]
                            n184 = Array Size(array=w539) -> (size(s)=w543:i32)
                            n185 = Decrement(x=w543) -> (x-1=w547:i32)
                            n186 = Index Array(array=w539, index=w547) -> (element=w544:T12)
                            n187 = Equal?(x=w540, y=w547) -> (x = y?=w545:bool)
                            n188 = Equal?(x=w538, y=w544) -> (x = y?=w546:bool)
                            n189 = And(x=w546, y=w545) -> (x .and. y?=w541:bool)
                          }
                          frame "lockin" {
                            n190 = local read "Config. fotodiodo y potenciometro"() -> (w569:T5)
                            n191 = Unbundle By Name(w569) -> ("tiempo. lect."=w568:i32, "num. med"=w567:i32, "usar multimetro"=w571:bool)
                            n192 = call "controllockin.vi"("usar multimetro"=w571, "Enum"=T11."Lockin", "num lecturas lockin"=w567, "tiempo lecturas lockin"=w568) -> ("multimetro"=w566:dbl, "Valor Lockin"=w565:dbl)  [unwired: 5 in, 1 out]
                            n193 = call "corr.vi"("Enum"=w573, "Orden"=w572, "Numeric"=w574) -> ("Enum 2"=w576:T12)  [unwired: 8 in]
                            n194 = Array Size(array=w572) -> (size(s)=w581:i32)
                            n195 = Decrement(x=w581) -> (x-1=w577:i32)
                            n196 = Index Array(array=w572, index=w577) -> (element=w580:T12)
                            n197 = Equal?(x=w574, y=w577) -> (x = y?=w579:bool)
                            n198 = Equal?(x=w573, y=w580) -> (x = y?=w578:bool)
                            n199 = And(x=w578, y=w579) -> (x .and. y?=w575:bool)
                          }
                          frame "laser" {
                            n200 = local read "Laser"() -> (w586:T4)
                            n201 = Unbundle By Name(w586) -> ("temperatura"=w585:dbl)
                            n202 = call "itc4000.vi"("Temperatura"=w585, "Corriente"=w584) -> ("Temperatura sal"=→"temperatura":dbl, "Corriente sal"=→"corriente laser":dbl)  [unwired: 7 in, 1 out]
                            n203 = call "corr.vi"("Enum"=w587, "Orden"=w588, "Numeric"=w589) -> ("Enum 2"=w591:T12)  [unwired: 8 in]
                            n204 = Array Size(array=w588) -> (size(s)=w596:i32)
                            n205 = Decrement(x=w596) -> (x-1=w592:i32)
                            n206 = Index Array(array=w588, index=w592) -> (element=w595:T12)
                            n207 = Equal?(x=w589, y=w592) -> (x = y?=w594:bool)
                            n208 = Equal?(x=w587, y=w595) -> (x = y?=w593:bool)
                            n209 = And(x=w593, y=w594) -> (x .and. y?=w590:bool)
                          }
                          frame "ninguno" {
                            n210 = call "corr.vi"("Enum"=w598, "Orden"=w597, "Numeric"=w599) -> ("Enum 2"=w601:T12)  [unwired: 8 in]
                            n211 = Array Size(array=w597) -> (size(s)=w602:i32)
                            n212 = Decrement(x=w602) -> (x-1=w606:i32)
                            n213 = Index Array(array=w597, index=w606) -> (element=w603:T12)
                            n214 = Equal?(x=w599, y=w606) -> (x = y?=w604:bool)
                            n215 = Equal?(x=w598, y=w603) -> (x = y?=w605:bool)
                            n216 = And(x=w605, y=w604) -> (x .and. y?=w600:bool)
                          }
                        }
                        n217 = Index Array(array="Gráficas visibles", index=5) -> (element=w436:bool)
                        n218 = property on="espectro" class="XYGraph (strict)"("Visible"=w436) -> ()  [unwired: 2 in, 2 out]
                        n219 = Index Array(array="Gráficas visibles", index=0) -> (element=w464:bool)
                        n220 = property on="Gráfica general" class="XYGraph (strict)"("Visible"=w464) -> ()  [unwired: 2 in, 2 out]
                        n221 = Index Array(array="Gráficas visibles", index=1) -> (element=w460:bool)
                        n222 = property on="Power meter" class="XYGraph (strict)"("Visible"=w460) -> ()  [unwired: 2 in, 2 out]
                        n223 = Index Array(array="Gráficas visibles", index=2) -> (element=w465:bool)
                        n224 = property on="I-V" class="XYGraph (strict)"("Visible"=w465) -> ()  [unwired: 2 in, 2 out]
                        n225 = Index Array(array="Gráficas visibles", index=3) -> (element=w441:bool)
                        n226 = Increment(x=w454) -> (x+1=w455:i32)
                        n227 = Wait (ms)(milliseconds to wait=u32 50) -> ()  [unwired: 1 out]
                        n228 = property on="multímetro" class="XYGraph (strict)"("Visible"=w441) -> ()  [unwired: 2 in, 2 out]
                        n229 = Index Array(array="Gráficas visibles", index=4) -> (element=w439:bool)
                        n230 = property on="division" class="XYGraph (strict)"("Visible"=w439) -> ()  [unwired: 2 in, 2 out]
                      }
                      n231 = local write "I 3"(w301) -> ()
                      n232 = local read "Config. fotodiodo y potenciometro"() -> (w305:T5)
                      n233 = local read "corriente"() -> (w302:dbl)
                      n234 = call "corrector.vi"("Array"=w335) -> ("valor salida"=w333:dbl)  [unwired: 10 in]
                      n235 = Build Array (concatenate)(w334, w333) -> (w332:dbl[])
                      n236 = local read "Orden"() -> (w310:T1)
                      n237 = call "sTRING2.vi"("angulo"=w316, "Orden"=w310, "Valor del voltaje"=w308, "cadena entrada"=w315, "corriente"=w314) -> ("String"=w304:string)  [unwired: 6 in]
                      n238 = Build Array (concatenate)(w352, w302) -> (w331:dbl[])
                      n239 = local read "Guardado"() -> (w298:bool)
                      n240 = call "corrector.vi"("Array"=w348) -> ("valor salida"=w349:dbl)  [unwired: 10 in]
                      "valor potenciometro" <- w349
                      n241 = Build Array (concatenate)(w351, w349) -> (w330:dbl[])
                      n242 = Unbundle By Name(w305) -> ("usar multimetro"=w306:bool)
                      n243 = call "corrector.vi"("Array"=w347) -> ("valor salida"=w343:dbl)  [unwired: 10 in]
                      "LockIn" <- w343
                      n244 = Build Array (concatenate)(w350, w343) -> (w312:dbl[])
                      n245 = call "corrector.vi"("Array"=w346) -> ("valor salida"=w345:dbl)  [unwired: 10 in]
                      n246 = Build Array (concatenate)(w353, w345) -> (w313:dbl[])
                      n247 = call "localizador.vi"("Orden"=w310) -> ("Tipo de Medición"=w309:T11, "Enum"=w303:T12)  [unwired: 9 in]
                      n248 = case shown="True" w298 {
                        tunnel: w304 -> [_ w364]
                        tunnel: w306 -> [_ w363]
                        tunnel: w303 -> [_ w360]
                        tunnel: w300 -> [w355 w357]
                        tunnel: [w355 w356] -> w299
                        frame False {
                        }
                        frame True {
                          n249 = local read "Nombre  archivo"() -> (w361:string)
                          n250 = local read "espectro aeereglo"() -> (w362:dbl[][])
                          n251 = local read "Orden"() -> (w359:T1)
                          n252 = call "buscarCCD.vi"("Orden"=w359) -> ("ccd?"=w358:bool)  [unwired: 9 in, 1 out]
                          n253 = case shown="True" w358 {
                            tunnel: w364 -> [_ _]
                            tunnel: w363 -> [_ _]
                            tunnel: w362 -> [_ w367]
                            tunnel: w361 -> [_ w389]
                            tunnel: w360 -> [_ _]
                            tunnel: w357 -> [w365 w390]
                            tunnel: [w365 w387] -> w356
                            frame False {
                            }
                            frame True {
                              (unwired) 2 ("index")
                              w388 = T1 [enum."CCD"] items=["espejos", "polarizador", "voltaje", "potenciometro ", "CCD", "lockin", "laser", "ninguno"] ("Orden")
                              n254 = local read "I 3"() -> (w382:i32)
                              n255 = local read "Orden"() -> (w386:T1)
                              n256 = local read "D 4"() -> (w383:i32)
                              n257 = local read "I 1"() -> (w381:i32)
                              n258 = local read "D 1"() -> (w385:i32)
                              n259 = local read "I 2"() -> (w380:i32)
                              n260 = local read "D 3"() -> (w384:i32)
                              n261 = local read "D 2"() -> (w379:i32)
                              n262 = call "indices.vi"("corriente laser"=w383, "voltaje"=w384, "polarizador"=w379, "espejo"=w385, "indice 3"=w382, "indice 2"=w380, "indice 1"=w381, "Orden"=w386) -> ("INDICES 2"=w371:i32[], "dimensiones"=w378:i32[])  [unwired: 2 in]
                              n263 = Index Array(array=w378) -> (element=w374:i32)  [unwired: 1 in]
                              n264 = Index Array(array=w371) -> (element=w370:i32)  [unwired: 1 in]
                              n265 = Index Array(array=w378, index=1) -> (element=w373:i32)
                              n266 = Index Array(array=w371, index=1) -> (element=w369:i32)
                              n267 = Index Array(array=w378, index=2) -> (element=w375:i32)
                              n268 = Index Array(array=w371) -> (element=w368:i32)  [unwired: 1 in]
                              n269 = call "arreglos.vi"("Orden"=w388, "DISP 1"=w370, "Cluster DISP 1"=w390, "DISP 2"=w369, "DISP 3"=w368, "DISPLONG 1"=w374, "DISPLONG 2"=w373, "DISPLONG 3"=w375, "nombre"=w389, "CCD"=w367, "MULTIMETRO"=FALSE) -> ("disp 1"=w387:T14)  [unwired: 13 in, 3 out]
                            }
                          }
                        }
                      }
                      n270 = call "corrector.vi"("Array"=w344) -> ()  [unwired: 10 in, 1 out]
                      n271 = call "corrector.vi"("Array"=w321) -> ("valor salida"=w319:dbl)  [unwired: 10 in]
                      "multimetro" <- w319
                      n272 = Build Array (concatenate)(w320, w319) -> (w311:dbl[])
                      n273 = case shown="\"polarizador\"" w303 {
                        tunnel: w332 -> [_ w392 _ _]
                        tunnel: w312 -> [_ w401 w415 _]
                        tunnel: w313 -> [_ w397 w410 _]
                        tunnel: w331 -> [_ w391 w416 _]
                        tunnel: w330 -> [_ _ w414 _]
                        tunnel: w312 -> [_ w398 w412 _]
                        tunnel: w311 -> [_ w399 w411 _]
                        tunnel: w309 -> [_ _ w408 _]
                        frame "espejos", Default {
                        }
                        frame "polarizador" {
                          w396 = "Grados(°)" ("Y Scale.Name Label.Text")
                          n274 = Bundle(w392, w391) -> (w393:cluster{dbl[], dbl[]})  [unwired: 1 in]
                          n275 = local write "I-V"(w393) -> ()
                          n276 = Bundle(w392, w401) -> (w400:cluster{dbl[], dbl[]})  [unwired: 1 in]
                          n277 = local write "Gráfica general"(w400) -> ()
                          n278 = local read "Config. fotodiodo y potenciometro"() -> (w395:T5)
                          n279 = property on="multímetro" class="XYGraph (strict)"("XScale.NameLbl.Text"=w396) -> ()  [unwired: 2 in, 2 out]
                          n280 = property on="division" class="XYGraph (strict)"("XScale.NameLbl.Text"=w396) -> ()  [unwired: 2 in, 2 out]
                          n281 = property on="Gráfica general" class="XYGraph (strict)"("XScale.NameLbl.Text"=w396) -> ()  [unwired: 2 in, 2 out]
                          n282 = Unbundle By Name(w395) -> ("usar multimetro"=w394:bool)
                          n283 = case shown="True" w394 {
                            tunnel: w399 -> [_ w407]
                            tunnel: w397 -> [_ w404]
                            tunnel: w398 -> [_ w406]
                            frame False {
                            }
                            frame True {
                              n284 = call "DIVISION.vi"("r"=w406, "dr"=w407) -> ("dr/r"=w405:dbl[])  [unwired: 9 in]
                              n285 = Bundle(w404, w406) -> (w402:cluster{dbl[], dbl[]})  [unwired: 1 in]
                              n286 = Bundle(w404, "dr/r"=w405) -> (w403:cluster{dbl[], "dr/r":dbl[]})  [unwired: 1 in]
                              n287 = local write "Dr/r"(w403) -> ()
                              n288 = local write "multímetro"(w402) -> ()
                            }
                          }
                        }
                        frame "voltaje" {
                          w409 = "Voltaje(V)" ("Y Scale.Name Label.Text")
                          n289 = local read "Config. fotodiodo y potenciometro"() -> (w418:T5)
                          n290 = Bundle(w410, w416) -> (w417:cluster{dbl[], dbl[]})  [unwired: 1 in]
                          n291 = Unbundle By Name(w418) -> ("usar multimetro"=w413:bool)
                          n292 = local write "I-V"(w417) -> ()
                          n293 = case shown="\"Lockin-potenciometro\"" w408 {
                            tunnel: w410 -> [w427 w430 w434]
                            tunnel: w415 -> [w426 w431 _]
                            tunnel: w414 -> [_ w429 w433]
                            frame "Lockin", Default {
                              n294 = Bundle(w427, w426) -> (w425:cluster{dbl[], dbl[]})  [unwired: 1 in]
                              n295 = local write "Gráfica general"(w425) -> ()
                            }
                            frame "Lockin-potenciometro" {
                              n296 = Bundle(w430, w431) -> (w432:cluster{dbl[], dbl[]})  [unwired: 1 in]
                              n297 = local write "Gráfica general"(w432) -> ()
                              n298 = Bundle(w430, w429) -> (w428:cluster{dbl[], dbl[]})  [unwired: 1 in]
                              n299 = local write "Power meter"(w428) -> ()
                            }
                            frame "Potenciometro" {
                              n300 = Bundle(w434, w433) -> (w435:cluster{dbl[], dbl[]})  [unwired: 1 in]
                              n301 = local write "Power meter"(w435) -> ()
                            }
                          }
                          n302 = property on="Gráfica general" class="XYGraph (strict)"("XScale.NameLbl.Text"=w409) -> ()  [unwired: 2 in, 2 out]
                          n303 = property on="division" class="XYGraph (strict)"("XScale.NameLbl.Text"=w409) -> ()  [unwired: 2 in, 2 out]
                          n304 = property on="multímetro" class="XYGraph (strict)"("XScale.NameLbl.Text"=w409) -> ()  [unwired: 2 in, 2 out]
                          n305 = case shown="True" w413 {
                            tunnel: w412 -> [_ w423]
                            tunnel: w410 -> [_ w420]
                            tunnel: w411 -> [_ w422]
                            frame False {
                            }
                            frame True {
                              n306 = call "DIVISION.vi"("r"=w422, "dr"=w423) -> ("dr/r"=w421:dbl[])  [unwired: 9 in]
                              n307 = Bundle(w420, w422) -> (→"multímetro":cluster{dbl[], dbl[]})  [unwired: 1 in]
                              n308 = Bundle(w420, "dr/r"=w421) -> (→"Dr/r":cluster{dbl[], "dr/r":dbl[]})  [unwired: 1 in]
                            }
                          }
                        }
                        frame "potenciometro " {
                        }
                      }
                      n309 = local read "stop medición"() -> (w326:bool)
                      n310 = local read "Orden"() -> (w328:T1)
                      n311 = Index Array(array=w328, index=2) -> (element=w324:T12)
                    }
                    n312 = local read "Guardar"() -> (w214:bool)
                    n313 = case shown="True" w214 {
                      tunnel: w213 -> [_ w285]
                      tunnel: w204 -> [_ w278]
                      tunnel: w201 -> [_ w283]
                      tunnel: w200 -> [_ w282]
                      tunnel: w199 -> [_ w281]
                      tunnel: w198 -> [_ w279]
                      tunnel: w197 -> [_ w280]
                      tunnel: w212 -> [_ w276]
                      frame False {
                      }
                      frame True {
                        n314 = local read "Orden"() -> (w287:T1)
                        n315 = local read "Config. fotodiodo y potenciometro"() -> (w274:T5)
                        n316 = call "buscarCCD.vi"("Orden"=w287) -> ("Orden 2"=w286:T1)  [unwired: 9 in, 1 out]
                        n317 = Unbundle By Name(w274) -> ("usar multimetro"=w273:bool)
                        n318 = local read "Nombre  archivo"() -> (w284:string)
                        n319 = call "DIVISION.vi"("r"=w278, "dr"=w279) -> ("dr/r"=w277:dbl[])  [unwired: 9 in]
                        n320 = local read "medir corriente"() -> (w275:bool)
                        n321 = call "guardadoarchivocompleto2.vi"("nombre"=w284, "lockin"=w279, "multimetro"=w273, "titulo grupo"=w285, "voltaje"=w283, "potenciometro"=w281, "angulo"=w280, "division"=w277, "Enum"=w276, "Orden"=w286, "polarizador"=w280, "corriente"=w282, "multim."=w278, "guardar corriente"=w275) -> ()  [unwired: 2 in]
                      }
                    }
                    n322 = local read "Orden"() -> (w194:T1)
                    n323 = local read "I 2"() -> (w190:i32)
                    n324 = local read "I 1"() -> (w193:i32)
                    n325 = local read "I 3"() -> (w189:i32)
                    n326 = local read "D 4"() -> (w191:i32)
                    n327 = call "buscarCCD.vi"("Orden"=w194) -> ("Orden 2"=w188:T1)  [unwired: 9 in, 1 out]
                    n328 = local read "D 1"() -> (w196:i32)
                    n329 = local read "D 2"() -> (w192:i32)
                    n330 = local read "D 3"() -> (w195:i32)
                    n331 = call "indices.vi"("corriente laser"=w191, "voltaje"=w195, "polarizador"=w192, "espejo"=w196, "indice 3"=w189, "indice 2"=w190, "indice 1"=w193, "Orden"=w188) -> ("INDICES 2"=w186:i32[], "dimensiones"=w187:i32[])  [unwired: 2 in]
                    n332 = call "NUEVOARREGLO.vi"("INDICES 2"=w186, "dimensiones"=w187) -> ("INDICES 3"=w177:i32[], "dimensiones 2"=w185:i32[])  [unwired: 8 in]
                    n333 = Index Array(array=w185, index=2) -> (element=w182:i32)
                    n334 = Index Array(array=w185) -> (element=w181:i32)  [unwired: 1 in]
                    n335 = Index Array(array=w185, index=1) -> (element=w180:i32)
                    n336 = local read "Orden"() -> (w229:T1)
                    n337 = Index Array(array=w229, index=1) -> (element=w223:T12)
                    n338 = local read "stop medición"() -> (w224:bool)
                    n339 = local read "Config. fotodiodo y potenciometro"() -> (w171:T5)
                    n340 = Index Array(array=w177, index=2) -> (element=w174:i32)
                    n341 = Index Array(array=w177) -> (element=w176:i32)  [unwired: 1 in]
                    n342 = Index Array(array=w177, index=1) -> (element=w175:i32)
                    n343 = Unbundle By Name(w171) -> ("usar multimetro"=w170:bool)
                    n344 = case shown="True" "Guardado" {
                      tunnel: [w248 w272] -> w208
                      tunnel: [w249 w271] -> w207
                      tunnel: [w247 w252] -> w206
                      tunnel: w205 -> [w247 w251]
                      tunnel: w204 -> [_ w270]
                      tunnel: w203 -> [w249 w250]
                      tunnel: w202 -> [w248 w269]
                      tunnel: w201 -> [_ w268]
                      tunnel: w200 -> [_ w267]
                      tunnel: w199 -> [_ w266]
                      tunnel: w198 -> [_ w265]
                      tunnel: w197 -> [_ w264]
                      tunnel: w188 -> [_ w263]
                      tunnel: w182 -> [_ w262]
                      tunnel: w181 -> [_ w261]
                      tunnel: w180 -> [_ w260]
                      tunnel: w176 -> [_ w259]
                      tunnel: w175 -> [_ w258]
                      tunnel: w174 -> [_ w257]
                      tunnel: w173 -> [w246 w255]
                      tunnel: [w246 w254] -> w172
                      tunnel: w170 -> [_ w253]
                      frame False {
                      }
                      frame True {
                        n345 = local read "Nombre  archivo"() -> (w256:string)
                        n346 = call "arreglos.vi"("Orden"=w263, "DISP 1"=w259, "Cluster DISP 1"=w269, "DISP 2"=w258, "DISP 3"=w257, "DISPLONG 1"=w261, "Cluster DISP 2"=w250, "DISPLONG 2"=w260, "DISPLONG 3"=w262, "nombre"=w256, "CORRIENTE"=w267, "MULTIMETRO 2"=w270, "VOLTAJE"=w268, "ANGULO"=w264, "POTENCIOMETRO"=w266, "LOCKIN"=w265, "MULTIMETRO"=w253, "Cluster DISP 4"=w255, "Cluster DISP 3"=w251) -> ("disp 2"=w271:T14, "disp 1"=w272:T14, "disp 3"=w252:T14, "disp 4"=w254:T14)  [unwired: 5 in]
                      }
                    }
                  }
                  n347 = property on="Image Pixels (U8)" class="Arr (strict)"("Visible"=w128) -> ()  [unwired: 2 in, 2 out]
                  n348 = property on="espectro aeereglo" class="Arr (strict)"("Visible"=w128) -> ()  [unwired: 2 in, 2 out]
                  n349 = local read "stop medición"() -> (w137:bool)
                  n350 = local read "Orden"() -> (w140:T1)
                  n351 = Index Array(array=w140, index=0) -> (element=w135:T12)
                }
              }
              frame #1 {
                n352 = local read "Orden"() -> (w611:T1)
                n353 = Search 1D Array(1D array=w611, element=T12."voltaje") -> (index of element=w609:i32)  [unwired: 1 in]
                n354 = Not Equal?(x=w609, y=-1) -> (x != y?=w607:bool)
                n355 = One Button Dialog(message="Terminó la medición.") -> ()  [unwired: 1 in, 1 out]
                n356 = case shown="True" w607 {
                  frame False {
                  }
                  frame True {
                    n357 = local read "Config. voltaje y corriente"() -> (w617:T3)
                    n358 = Unbundle By Name(w617) -> ("VISA resource name"=w616:refnum<visa-resource-name>, "Function(0:Voltage)"=w615:u16)
                    n359 = call "fuenteVoltajenueva.vi"("entrada"=0.0, "Source Mode  (0: Voltage)"=w615, "VISA resource name"=w616) -> ("CORRIENTE"=w613:dbl, "VOLTAJE"=w614:dbl)  [unwired: 7 in]
                    n360 = local write "corriente"(w613) -> ()
                    n361 = local write "voltaje"(w614) -> ()
                  }
                }
              }
            }
          }
        }
        n362 = shared-variable "NI-cRIO9074\\Library_CRIO.lvlib\\Stop_read"("stop") -> ()  [unwired: 1 in, 1 out]
      }
    }
  }
